vi "Eval y=f(x1,x2) Prep.vi"(4 "End":dbl[](array[numeric]) format="%.2f", 6 "Start":dbl[](array[numeric]) format="%.2f", 7 "Variables":string[](array[string]), 8 "formula":string) -> (0 "time [msec]":u32, 1 "error (general)":bool, 2 "error situation 1":bool, 3 "formula copy":string, 5 "error situation 2":bool)   [LabVIEW 2017, in "NI_Gmath.lvlib"]
uses:
  <vilib>/gmath/NI_Gmath.lvlib
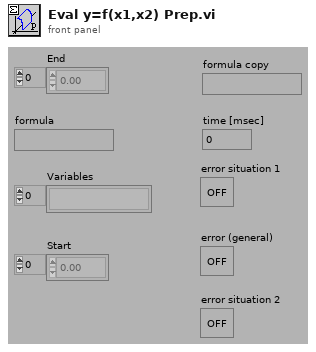
[diagram p1: front panel]
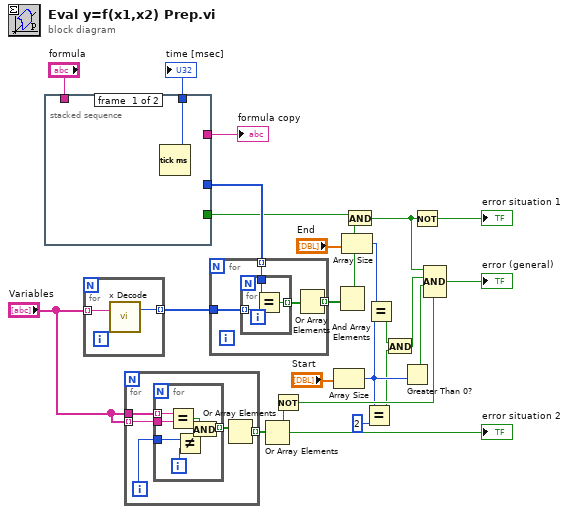
[diagram p0: block diagram]
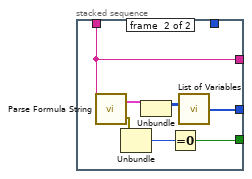
[diagram p2: hidden frame]
diagram:
  n1 = stacked-sequence {
    tunnel: [_ w32] -> w2
    tunnel: [w25 _] -> w4
    tunnel: [_ w31] -> w18
    tunnel: [_ w30] -> w3
    tunnel: "formula" -> [_ w30]
    frame #0 {
      n2 = Tick Count (ms)() -> (millisecond timer value=w25:u32)
    }
    frame #1 {
      n3 = call <vilib>:"Parse Formula String.vi"("formula"=w30) -> ("error out"=w29:errorcluster, "Parsed Formula"=w27:cluster{"Table":i32[][], "Y Values":dbl[]})  [unwired: 1 in]
      n4 = Unbundle(w29) -> ("code"=w28:i32)  [unwired: 2 out]
      n5 = Unbundle(w27) -> ("Table"=w26:i32[][])  [unwired: 1 out]
      n6 = Equal To 0?(x=w28) -> (x = 0?=w32:bool)
      n7 = call <vilib>:"List of Variables.vi"("Table"=w26) -> ("List of variables"=w31:i32[])
    }
  }
  "time [msec]" <- w4
  "formula copy" <- w3
  n8 = for {
    tunnel: "Variables" -> [w34] mode=indexing
    tunnel: [w33] -> w19 mode=indexing
    n9 = call <vilib>:"x Decode.vi"("x string"=w34) -> ("number"=w33:i32)  [unwired: 1 in, 1 out]
  }
  n10 = for {
    tunnel: "Variables" -> [w39]
    tunnel: "Variables" -> [w38] mode=indexing
    tunnel: [w35] -> w20 mode=indexing
    i -> [w37]
    n11 = for {
      tunnel: w39 -> [w46] mode=indexing
      tunnel: w38 -> [w45]
      tunnel: w37 -> [w44]
      tunnel: [w40] -> w36 mode=indexing
      i -> [w43]
      n12 = Equal?(x=w46, y=w45) -> (x = y?=w42:bool)
      n13 = Not Equal?(x=w44, y=w43) -> (x != y?=w41:bool)
      n14 = And(x=w42, y=w41) -> (x .and. y?=w40:bool)
    }
    n15 = Or Array Elements(Boolean array=w36) -> (logical OR=w35:bool)
  }
  n16 = for {
    tunnel: [w49] -> w17 mode=indexing
    tunnel: w18 -> [w48] mode=indexing
    tunnel: w19 -> [w47]
    n17 = for {
      tunnel: [w53] -> w50 mode=indexing
      tunnel: w48 -> [w52]
      tunnel: w47 -> [w51] mode=indexing
      n18 = Equal?(x=w52, y=w51) -> (x = y?=w53:bool)
    }
    n19 = Or Array Elements(Boolean array=w50) -> (logical OR=w49:bool)
  }
  n20 = Or Array Elements(Boolean array=w20) -> (logical OR=w21:bool)
  "error situation 2" <- w21
  n21 = Not(x=w21) -> (.not. x?=w23:bool)
  n22 = Array Size(array="Start") -> (size(s)=w11:i32)
  n23 = And Array Elements(Boolean array=w17) -> (logical AND=w1:bool)
  n24 = Array Size(array="End") -> (size(s)=w8:i32)
  n25 = And(x=w2, y=w1) -> (x .and. y?=w14:bool)
  n26 = Equal?(x=w11, y=2) -> (x = y?=w9:bool)
  n27 = Equal?(x=w8, y=w11) -> (x = y?=w10:bool)
  n28 = And(x=w10, y=w9) -> (x .and. y?=w13:bool)
  n29 = Greater Than 0?(x=w11) -> (x > 0?=w12:bool)
  n30 = Not(x=w14) -> (.not. x?=→"error situation 1":bool)
  n31 = Compound Arithmetic op=AND(w14, w13, w12, w23) -> (→"error (general)":bool)
